vi "MGI Round to Decimal Place.vi"(1 "Round (To Nearest)":T1, 2 "Decimal Digits":i32, 3 "Number":dbl format="%.12e") -> (0 "Rounded":dbl format="%.12e")   [LabVIEW 2016]
doc: "Rounds the input number to the specified number of decimal places. Note that some decimal numbers (like 0.1) cannot be exactly represented. For such numbers, the \"rounded\" number is only correct out to 13 decimal places.\n\nAuthored by Shawn Walpole\nsupport@mooregoodideas.com\nwww.mooregoodideas.com\n\nCopyright (c) 2010, Moore Good Ideas, Inc.\n\nAll rights reserved.\n\nRedistribution and use in source and binary forms, with or without modification, are permitted provided that the following conditions are met:\n\n * Redistributions of source code must retain the above copyright notice, this list of conditions and the following disclaimer.\n * Redistributions in binary form must reproduce the above copyright notice, this list of conditions and the following disclaimer in the documentation and/or other materials provided with the distribution.\n * Neither the name of Moore Good Ideas, Inc. nor the names of its contributors may be used to endorse or promote products derived from this software without specific prior written permission.\n\nTHIS SOFTWARE IS PROVIDED BY THE COPYRIGHT HOLDERS AND CONTRIBUTORS \"AS IS\" AND ANY EXPRESS OR IMPLIED WARRANTIES, INCLUDING, BUT NOT LIMITED TO, THE IMPLIED WARRANTIES OF MERCHANTABILITY AND FITNESS FOR A PARTICULAR PURPOSE ARE DISCLAIMED. IN NO EVENT SHALL THE COPYRIGHT OWNER OR CONTRIBUTORS BE LIABLE FOR ANY DIRECT, INDIRECT, INCIDENTAL, SPECIAL, EXEMPLARY, OR CONSEQUENTIAL DAMAGES (INCLUDING, BUT NOT LIMITED TO, PROCUREMENT OF SUBSTITUTE GOODS OR SERVICES; LOSS OF USE, DATA, OR PROFITS; OR BUSINESS INTERRUPTION) HOWEVER CAUSED AND ON ANY THEORY OF LIABILITY, WHETHER IN CONTRACT, STRICT LIABILITY, OR TORT (INCLUDING NEGLIGENCE OR OTHERWISE) ARISING IN ANY WAY OUT OF THE USE OF THIS SOFTWARE, EVEN IF ADVISED OF THE POSSIBILITY OF SUCH DAMAGE."
uses:
  <userlib>/_MGI/Numeric/Rounding/MGI Round to Decimal Place Enum.ctl
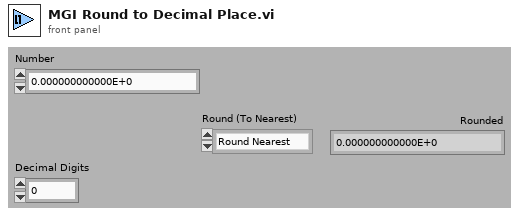
[diagram p1: front panel]
types:
  T1 = typedef "MGI Round to Decimal Place Enum.ctl" = enum16{"Round Nearest", "Round +Inf", "Round -Inf"}
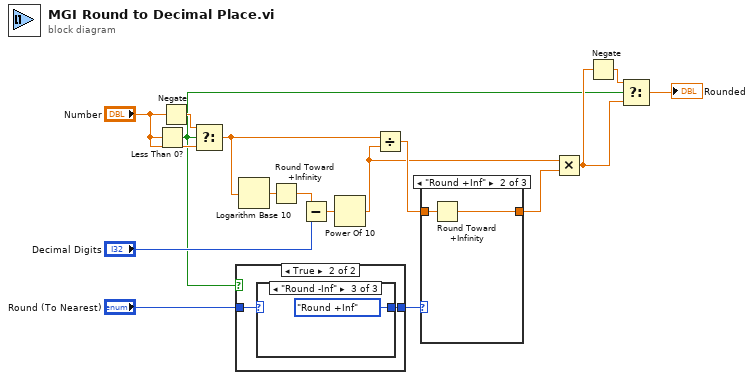
[diagram p0: block diagram]
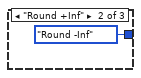
[diagram p4: hidden frame]
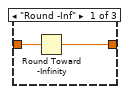
[diagram p5: hidden frame]
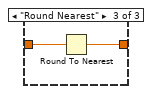
[diagram p6: hidden frame]
diagram:
  n1 = Less Than 0?(x="Number") -> (x < 0?=w3:bool)
  n2 = Negate(x="Number") -> (-x=w7:dbl)
  n3 = Select(t=w7, s=w3, f="Number") -> (s? t:f=w9:dbl)
  n4 = case shown="True" w3 {
    tunnel: "Round (To Nearest)" -> [w17 w19]
    tunnel: [w17 w18] -> w1
    frame False {
    }
    frame True {
      n5 = case shown="\"Round -Inf\"" w19 {
        selector: w19 -> [w20 _ _]
        tunnel: [w20 MGI_Round_to_Decimal_Place_Enum."Round -Inf" ("Round (To Nearest)") MGI_Round_to_Decimal_Place_Enum."Round +Inf" ("Round (To Nearest)")] -> w18
        frame "Round Nearest" {
        }
        frame "Round +Inf" {
        }
        frame "Round -Inf" {
        }
      }
    }
  }
  n6 = Logarithm Base 10(1:w9) -> (0:w15:dbl)
  n7 = Round Toward +Infinity(x=w15) -> (ceil(x): smallest int >= x=w14:dbl)
  n8 = Subtract(x=w14, y="Decimal Digits") -> (x-y=w13:dbl)
  n9 = Power Of 10(x=w13) -> (10^x=w10:dbl)
  n10 = Divide(x=w9, y=w10) -> (x/y=w12:dbl)
  n11 = case shown="\"Round +Inf\"" w1 {
    tunnel: w12 -> [w24 w26 w28]
    tunnel: [w23 w25 w27] -> w11
    frame "Round -Inf" {
      n12 = Round Toward -Infinity(1:w24) -> (0:w23:dbl)
    }
    frame "Round +Inf" {
      n13 = Round Toward +Infinity(x=w26) -> (ceil(x): smallest int >= x=w25:dbl)
    }
    frame "Round Nearest" {
      n14 = Round To Nearest(number=w28) -> (nearest integer value=w27:dbl)
    }
  }
  n15 = Multiply(x=w10, y=w11) -> (x*y=w5:dbl)
  n16 = Negate(x=w5) -> (-x=w6:dbl)
  n17 = Select(t=w6, s=w3, f=w5) -> (s? t:f=→"Rounded":dbl)
